vi "Uno.vi"() -> ()   [LabVIEW 2026]
panel:
  in  "Pin":u8=4 min=4 max=40
  in  "Estado":bool
  in  "Stop Button":bool
  in  "VISA resource name":refnum<visa-resource-name>
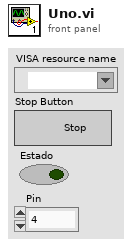
[diagram p1: front panel]
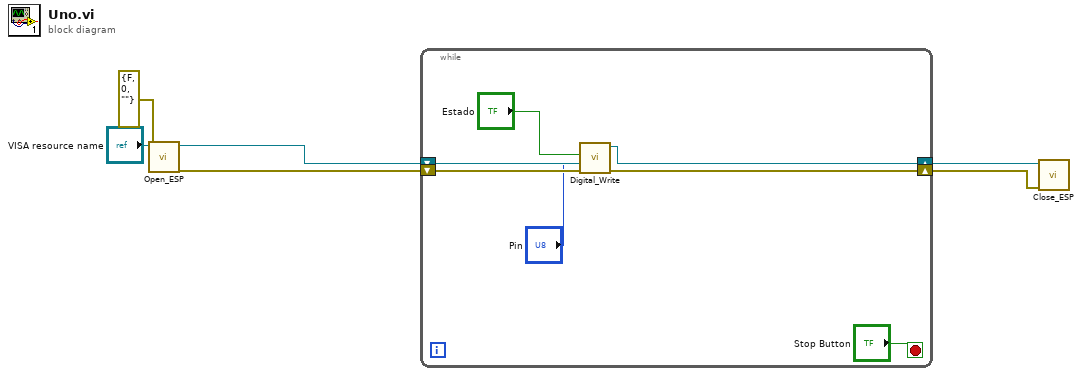
[diagram p0: block diagram]
diagram:
  n1 = call "Open_ESP.vi"("error in (no error)"=errorcluster {"status"=FALSE, "code"=0, "source"=""}, "VISA resource name"="VISA resource name") -> ("error out"=w1:errorcluster, "VISA resource name out"=w4:refnum<visa-resource-name>)  [unwired: 8 in]
  n2 = while {
    shift-right: [w12] -> w3
    shift-left: w4 -> [w13]
    shift-right: [w11] -> w2
    shift-left: w1 -> [w10]
    stop <- "Stop Button" stop-if-true
    n3 = call "Digital_Write.vi"("error in (no error)"=w10, "Pin"="Pin", "Estado"="Estado", "VISA resource name"=w13) -> ("error out"=w11:errorcluster, "VISA resource name out"=w12:refnum<visa-resource-name>)  [unwired: 6 in]
  }
  n4 = call "Close_ESP.vi"("error in (no error)"=w2, "VISA resource name"=w3) -> ()  [unwired: 9 in, 1 out]
